vi "Vision Research Phantom Series Close.vi"(5 "Error In (no error)":errorcluster) -> (19 "Error Out":errorcluster)   [LabVIEW 2013, in "VRI.lvlib"]
doc: "This VI closes the reference to the Vision Research Phantom Series camera. This VI executes when an error is passed in.\n\nWritten by:\nBLOOMY CONTROLS, INC\nWINDSOR, CT 06095, USA\n860-298-9925\nwww.bloomy.com\nV1.0.0\nMay, 2004"
uses:
  VRI.lvlib
  Phantom DLLs/PhCon.Dll
panel:
  out "HRESULT":i32
  # "For instructions on the use of this VI, press Ctrl+H to display the help window and move the mouse over the icon, controls, and indicators"
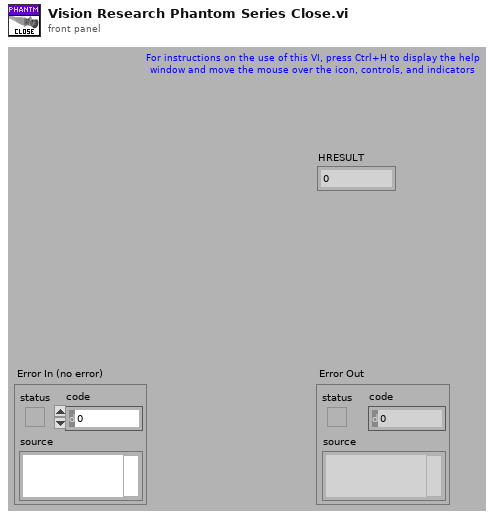
[diagram p1: front panel]
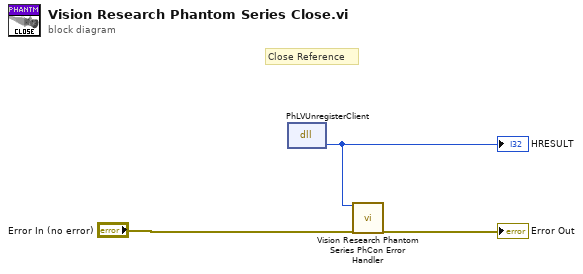
[diagram p0: block diagram]
diagram:
  # "Close Reference"
  n1 = dll-call lib="C:/Projects/SDK/64-bit/Vision Research Phantom Series Labview Driver/Phantom DLLs/PhCon.dll" fn="PhLVUnregisterClient"() -> (w1:i32)  [unwired: 3 in, 2 out]
  "HRESULT" <- w1
  n2 = call "Vision Research Phantom Series PhCon Error Handler.vi"("ErrNo"=w1, "Error In (no error)"="Error In (no error)") -> ("Error Out"=→"Error Out":errorcluster)  [unwired: 17 out]
